vi "fpga main.vi"() -> ()   [LabVIEW 2017]
uses:
  <vilib>/rvi/interface/nirviMethod/nirviMethod.xnode
  <vilib>/rvi/interface/nirviReadWriteControl/nirviReadWriteControl.xnode
  <vilib>/rvi/interface/nirviOpenFPGA/nirviOpenFPGA.xnode
  <vilib>/FPGAPlugInAG/Dynamic/niLvFpga_Run_Dynamic.vi
  <vilib>/FPGAPlugInAG/Dynamic/niLvFpga_Abort_Dynamic.vi
  <vilib>/platform/TimedLoop/XDataNode/XDataNode.xnode
  <vilib>/Platform/TimedLoop/XDataNode/nitl_modes.ctl
  <vilib>/Platform/TimedLoop/XDataNode/XDNodeRunTimeDep.lvlib
  <vilib>/Platform/TimedLoop/XDataNode/wakeup.ctl
  <vilib>/Platform/TimedLoop/XDataNode/timing_clust.ctl
  <vilib>/rvi/interface/Simulation/niFpgaSimulationCallBeginRW.vi
  <vilib>/rvi/errors/niLvFpgaAdjustHostInterfaceError.vi
  FPGA Bitfiles/fpgaproject_FPGATarget_fpgamain2_gPNnZPUgBMY.lvbitx
  fpga main2.vi
  <vilib>/FPGAPlugInAG/Dynamic/niLvFpga_StartFifo_Dynamic.vi
  <vilib>/rvi/errors/niLvFpgaMergeErrorWithErrorCode.vi
panel:
  in  "time format string (%c)":string
  out "size(s)":i32[](array[numeric])
  in  "Period":i64
  out "Encoder Position":dbl format="%#_8g"
  in  "Position Reset":bool
  out "Array 2":string[][](array[string])
  out "速率":dbl
  out "Real period":u32
  out "error out 3":errorcluster
  out "error out 2":errorcluster
  out "error out":errorcluster
  in  "stop":bool
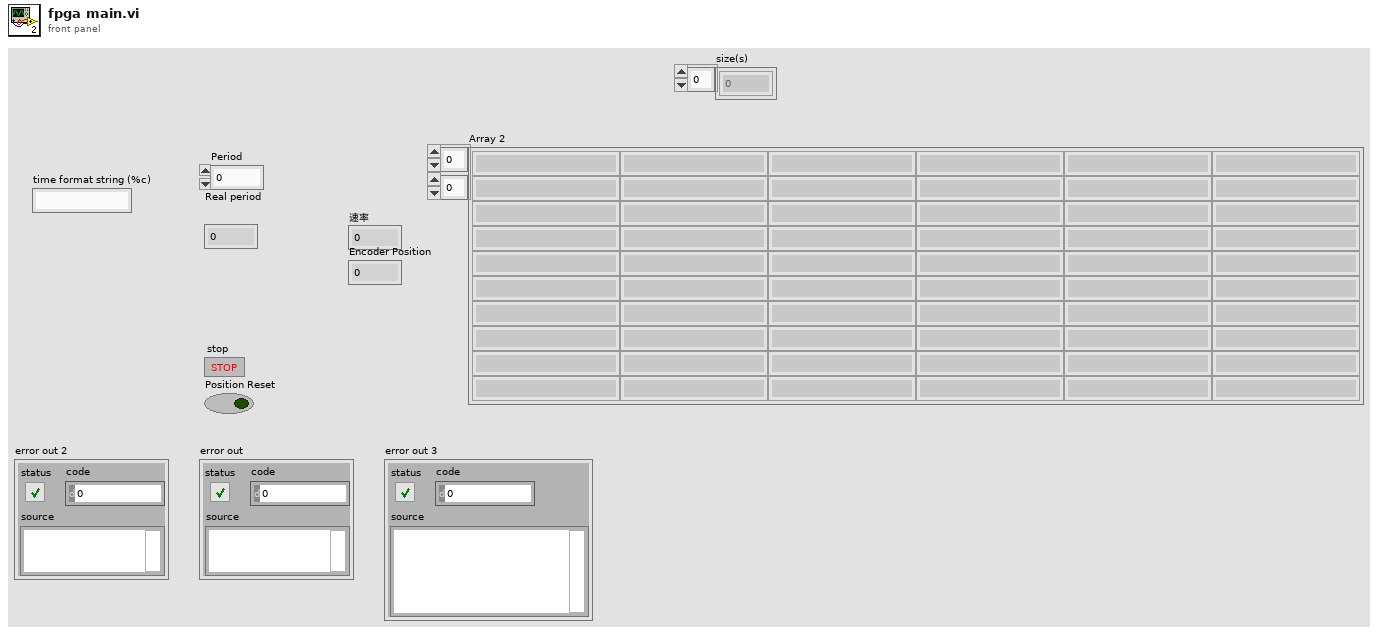
[diagram p1: front panel]
types:
  T1 = enum16{"open", "replace", "create", "open or create", "replace or create", "replace or create with confirmation"}
  T2 = typedef "XDNodeRunTimeDep.lvlib/timing_clust.ctl" = cluster{"Expected End [f-1]":u64, "Actual End [f-1]":u64, "Finished Late? [f-1]":bool, "Expected End [i-1]":u64, "Actual End [i-1]":u64, "Finished Late? [i-1]":bool, "Expected Start [i]":u64, "Actual Start [i]":u64, "Expected Start [f]":u64, "Actual Start [f]":u64, "Source Name":string, "Structure Name":string, "Period":i64, "Deadline":i64, "Offset":i64, "Start":i64, "Priority":i32, "Timeout":i32, "Mode":T3, "Wakeup Reason":T4, "Error":errorcluster, "Source Type":string, "Secondary Source Type":string, "Global End Time":u64, "Global Start Time":u64, "Frame Duration":u64, "Iteration Duration":u64, "Assigned CPU":i32, "I/O Scan Engine Mode":u32}
  T3 = typedef "XDNodeRunTimeDep.lvlib/nitl_modes.ctl" = enum32{"No Change", "Process missed periods, maintain original phase", "Discard missed periods, maintain original phase", "Process missed periods, ignore original phase", "Discard missed periods, ignore original phase"}
  T4 = typedef "XDNodeRunTimeDep.lvlib/wakeup.ctl" = enum32{"Normal", "Aborted", "Asynchronous wakeup", "Timing source error", "Timed loop error", "Timeout"}
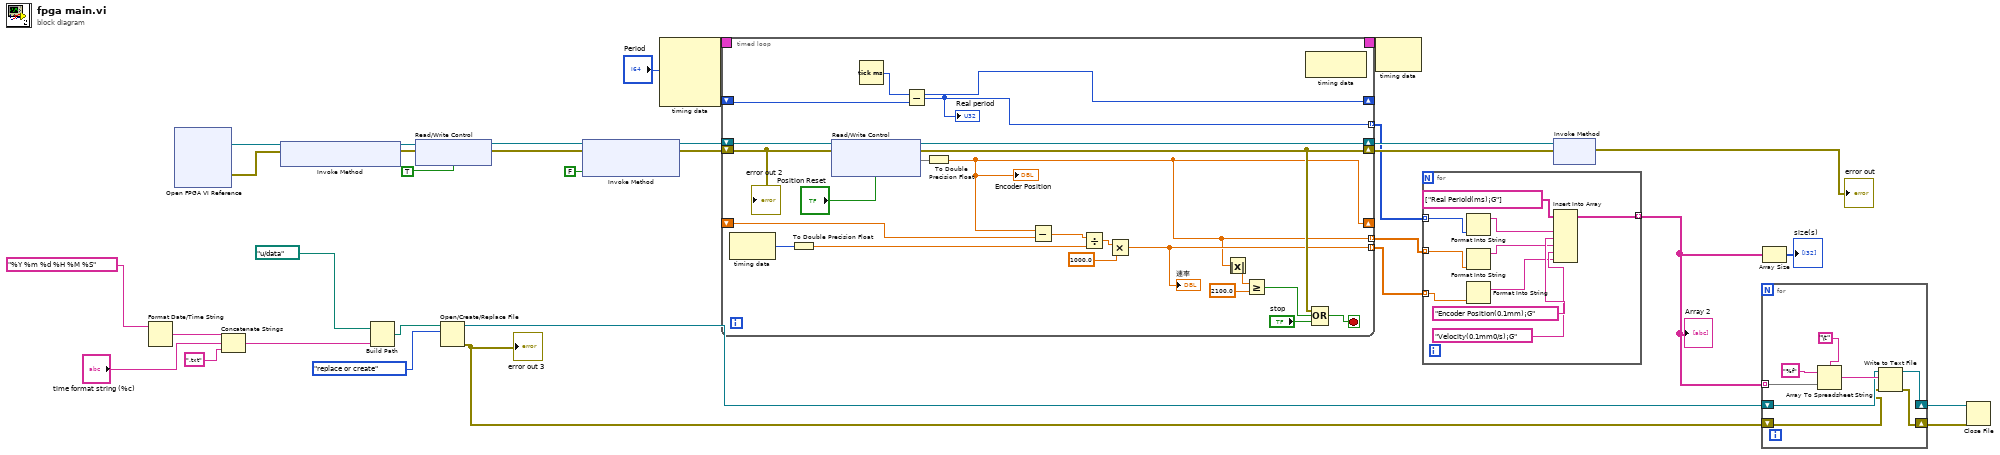
[diagram p0: block diagram]
diagram:
  n1 = Format Date/Time String(time format string (%c)="%Y %m %d %H %M %S") -> (date/time string=w26:string)  [unwired: 2 in]
  n2 = xnode "Open FPGA VI Reference"() -> ("FPGA VI Reference Out"=w12:refnum<k20>, "error out"=w11:errorcluster)  [unwired: 2 in]
  n3 = Concatenate Strings(w26, "time format string (%c)", ".txt" ("string")) -> (w25:string)
  n4 = xnode "Invoke Method"("FPGA VI Reference In"=w12, "error in"=w11) -> ("FPGA VI Reference Out"=w14:refnum<k20>, "error out"=w13:errorcluster)
  n5 = Build Path(base path=path "u:/data", name or relative path=w25) -> (appended path=w24:path)
  n6 = xnode "Read/Write Control"("FPGA VI Reference In"=w14, "error in"=w13, "Position Reset"=TRUE) -> ("FPGA VI Reference Out"=w29:refnum<k20>, "error out"=w28:errorcluster)
  n7 = Open/Create/Replace File(file path (use dialog)=w24, operation (0:open)=T1."replace or create") -> (refnum out=w22:refnum<file>, error out=w21:errorcluster)  [unwired: 4 in, 1 out]
  "error out 3" <- w21
  n8 = xnode "Invoke Method"("FPGA VI Reference In"=w29, "error in"=w28, "Wait Until Done (F)"=FALSE) -> ("FPGA VI Reference Out"=w31:refnum<k20>, "error out"=w30:errorcluster)
  n9 = node-c288("Period") -> (w17:T2)  [unwired: 3 in]
  n10 = timed-loop {
    shift-right: [w50] -> w33
    shift-left: w31 -> [w48]
    shift-right: [w43] -> w32
    shift-left: w30 -> [w51]
    shift-right: [w54] -> _
    shift-left: _ -> [w55]
    timing: w17 -> [_]
    timing-out: [_] -> w16
    tunnel: [w53] -> w9 mode=indexing
    shift-right: [w34] -> _
    shift-left: _ -> [w49]
    tunnel: [w34] -> w10 mode=indexing
    tunnel: [w36] -> w7 mode=indexing
    stop <- w45 stop-if-true
    n11 = node-c288() -> (w39:i64)  [unwired: 1 in]
    n12 = To Double Precision Float(number=w39) -> (double precision float=w38:dbl)
    n13 = xnode "Read/Write Control"("FPGA VI Reference In"=w48, "error in"=w51, "Position Reset"="Position Reset") -> ("FPGA VI Reference Out"=w50:refnum<k20>, "error out"=w43:errorcluster, "Position (Counts)"=w40)
    n14 = Tick Count (ms)() -> (millisecond timer value=w54:u32)
    n15 = Subtract(x=w54, y=w55) -> (x-y=w53:u32)
    "Real period" <- w53
    n16 = To Double Precision Float(number=w40) -> (double precision float=w34:dbl)
    "Encoder Position" <- w34
    n17 = Subtract(x=w34, y=w49) -> (x-y=w52:dbl)
    n18 = Divide(x=w52, y=w38) -> (x/y=w37:dbl)
    n19 = Multiply(x=w37, y=1000.0) -> (x*y=w36:dbl)
    "速率" <- w36
    n20 = Absolute Value(x=w34) -> (abs(x)=w35:dbl)
    n21 = Greater Or Equal?(x=w35, y=2100.0) -> (x >= y?=w42:bool)
    n22 = node-c288() -> ()  [unwired: 1 in, 1 out]
    n23 = Compound Arithmetic op=OR(w43, w42, "stop") -> (w45:bool)
    "error out 2" <- w51
  }
  n24 = node-c288(w16) -> ()  [unwired: 1 out]
  n25 = for {
    tunnel: [w66] -> w5 mode=indexing
    tunnel: w10 -> [w63] mode=indexing
    tunnel: w9 -> [w61] mode=indexing
    tunnel: w7 -> [w65] mode=indexing
    n26 = Format Into String(w61) -> (resulting string=w60:string)  [unwired: 3 in, 1 out]
    n27 = Format Into String(w63) -> (resulting string=w62:string)  [unwired: 3 in, 1 out]
    n28 = Format Into String(w65) -> (resulting string=w64:string)  [unwired: 3 in, 1 out]
    n29 = Insert Into Array(array=string[] ["Real Periold(ms)¡G"], new element #1=w60, new element #2="Encoder Position(0.1mm)¡G", new element #3=w62, new element #4="Velocity(0.1mm0/s)¡G", new element #5=w64) -> (w66:string[])  [unwired: 1 in]
  }
  "Array 2" <- w5
  n30 = xnode "Invoke Method"("FPGA VI Reference In"=w33, "error in"=w32) -> ("error out"=→"error out":errorcluster)  [unwired: 1 out]
  n31 = for {
    shift-right: [w70] -> w19
    shift-left: w22 -> [w73]
    shift-right: [w71] -> w20
    shift-left: w21 -> [w72]
    tunnel: w5 -> [w69] mode=indexing
    n32 = Array To Spreadsheet String(delimiter (Tab)="\t", array=w69, 3:"%f" ("format string")) -> (spreadsheet string=w74:string)
    n33 = Write to Text File(file (use dialog)=w73, text=w74, error in=w72) -> (refnum out=w70:refnum<file>, error out=w71:errorcluster)  [unwired: 1 in, 1 out]
  }
  n34 = Array Size(array=w5) -> (size(s)=→"size(s)":i32[])
  n35 = Close File(refnum=w19, error in=w20) -> ()  [unwired: 2 out]
